vi "Fuzzy_Output.vi"() -> ()   [LabVIEW 2016]
panel:
  in  "OK Button":bool
  in  "stop":bool
  in  "Membership Function 3":dbl[](array[numeric])
  in  "Membership Function 2":dbl[](array[numeric])
  in  "Membership Function 1":dbl[](array[numeric])
  out "XY Graph":cluster{"Array":dbl[], dbl[]}[](graph)
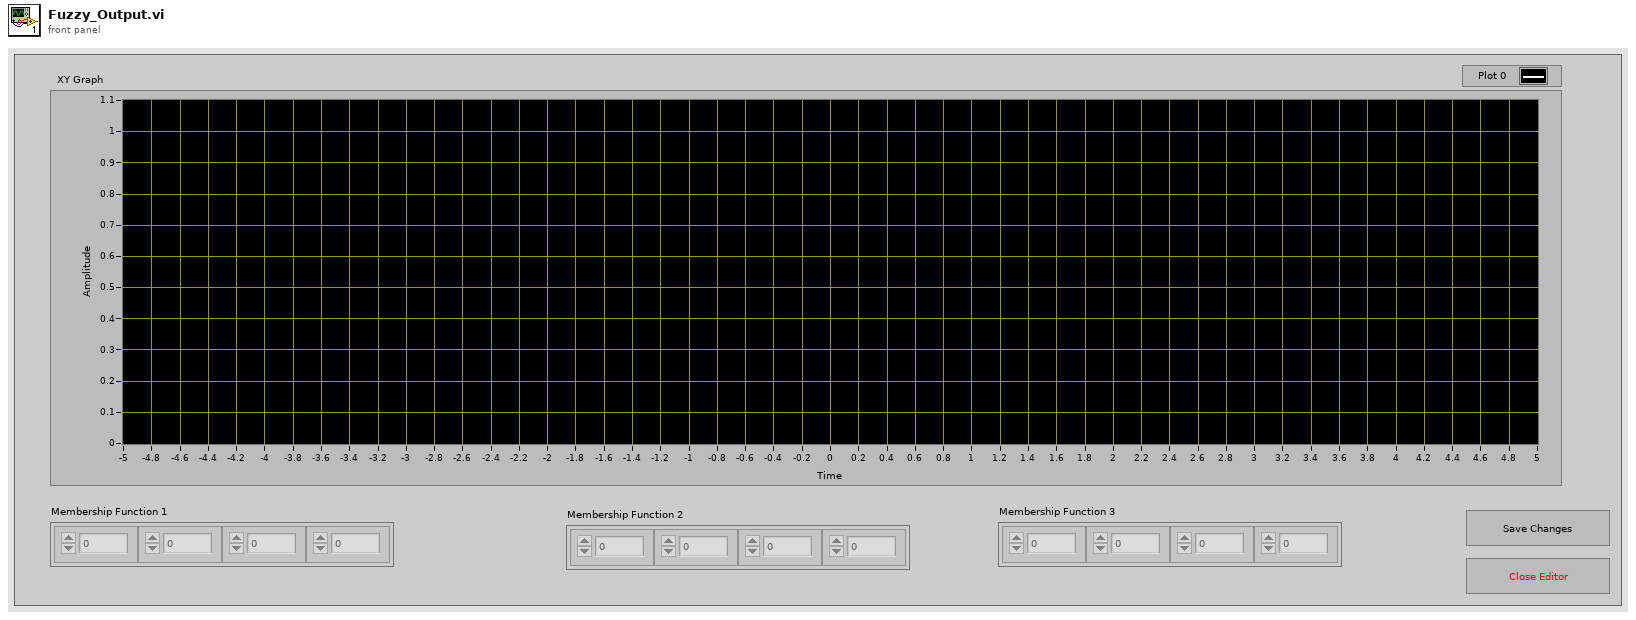
[diagram p1: front panel]
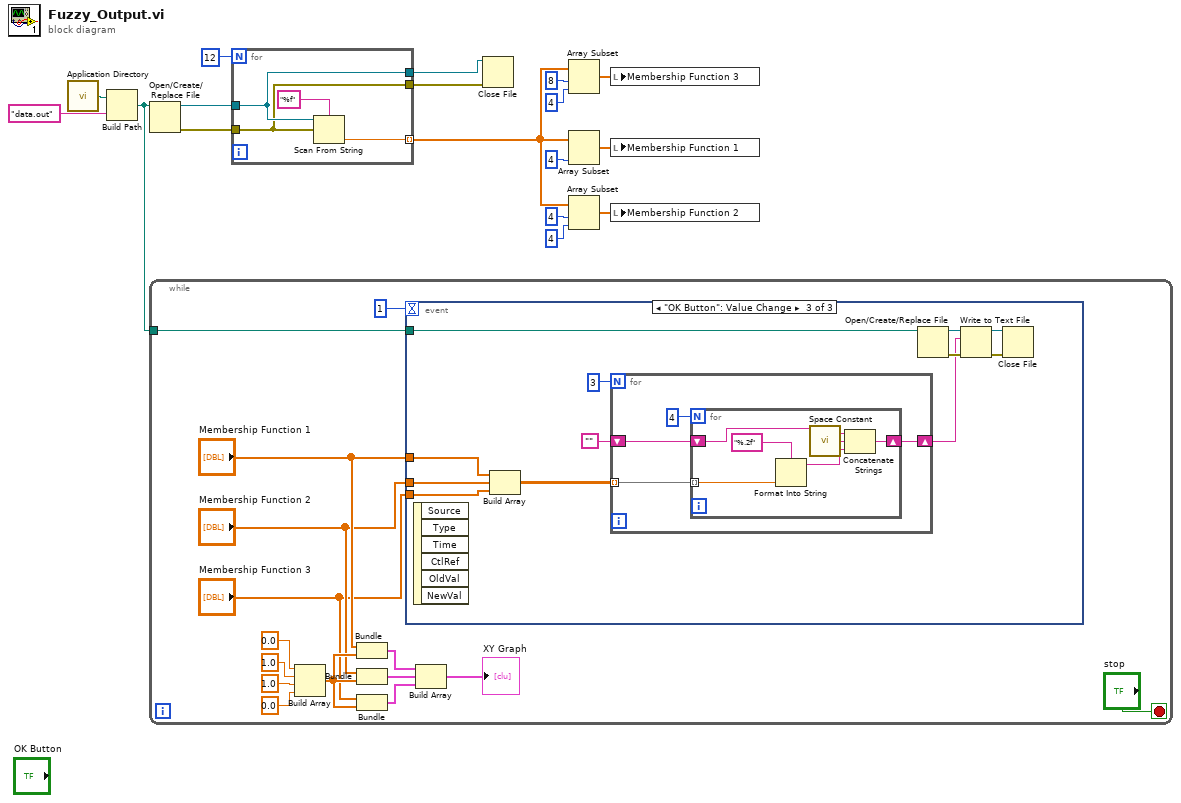
[diagram p0: block diagram]
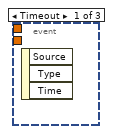
[diagram p2: hidden frame]
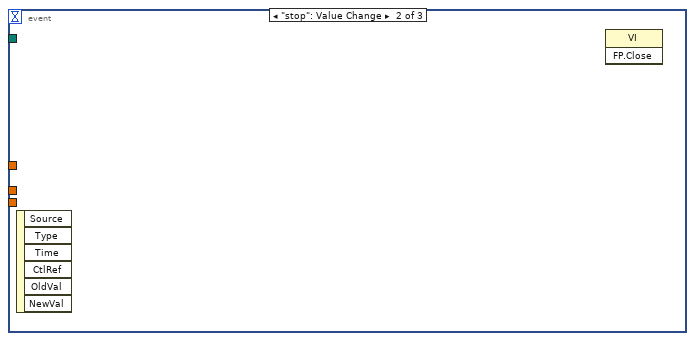
[diagram p3: hidden frame]
diagram:
  n1 = call <vilib>:"Application Directory.vi"() -> ("Application Directory"=w16:path)
  n2 = Build Path(base path=w16, name or relative path="data.out") -> (appended path=w1:path)
  n3 = Open/Create/Replace File(file path (use dialog)=w1) -> (refnum out=w14:refnum<file>, error out=w13:errorcluster)  [unwired: 5 in, 1 out]
  n4 = while {
    tunnel: w1 -> [w18]
    stop <- "stop" stop-if-true
    n5 = Build Array(0.0 ("element"), 1.0 ("element"), 1.0 ("element"), 0.0 ("element")) -> (w24:dbl[])
    n6 = Bundle("Membership Function 1"="Membership Function 1", w24) -> (w32:cluster{"Membership Function 1":dbl[], dbl[]})  [unwired: 1 in]
    n7 = Bundle("Membership Function 2"="Membership Function 2", w24) -> (w31:cluster{"Membership Function 2":dbl[], dbl[]})  [unwired: 1 in]
    n8 = Bundle("Membership Function 3"="Membership Function 3", w24) -> (w30:cluster{"Membership Function 3":dbl[], dbl[]})  [unwired: 1 in]
    n9 = event shown="[2] \"OK Button\": Value Change" {
      selector: _ -> [_ _ _]
      dyn-events: _ -> [_ _ _]
      timeout: 1 -> [_ _ _]
      tunnel: "Membership Function 1" -> [_ _ w36]
      tunnel: "Membership Function 2" -> [_ _ w35]
      tunnel: "Membership Function 3" -> [_ _ w34]
      tunnel: w18 -> [_ _ w33]
      event Timeout {
        n10 = event-data() -> ()  [unwired: 1 in, 3 out]
      }
      event "stop": Value Change {
        n11 = event-data() -> ()  [unwired: 1 in, 6 out]
        n12 = invoke class="VI" method="FP.Close"() -> ()  [unwired: 3 in, 3 out]
      }
      event "OK Button": Value Change {
        n13 = event-data() -> ()  [unwired: 1 in, 6 out]
        n14 = Build Array(w36, w35, w34) -> (w38:dbl[][])
        n15 = for {
          N: 3 -> [_]
          tunnel: w38 -> [w47] mode=indexing
          shift-right: [w46] -> w40
          shift-left: "" -> [w45]
          n16 = for {
            N: 4 -> [_]
            tunnel: w47 -> [w49] mode=indexing
            shift-right: [w53] -> w46
            shift-left: w45 -> [w52]
            n17 = Format Into String(format string="%.2f", w49) -> (resulting string=w50:string)  [unwired: 2 in, 1 out]
            n18 = call <vilib>:"Space Constant.vi"() -> ("String"=w51:string)
            n19 = Concatenate Strings(w52, w51, w50) -> (w53:string)
          }
        }
        n20 = Open/Create/Replace File(file path (use dialog)=w33) -> (refnum out=w41:refnum<file>, error out=w42:errorcluster)  [unwired: 5 in, 1 out]
        n21 = Write to Text File(file (use dialog)=w41, text=w40, error in=w42) -> (refnum out=w43:refnum<file>, error out=w44:errorcluster)  [unwired: 1 in, 1 out]
        n22 = Close File(refnum=w43, error in=w44) -> ()  [unwired: 2 out]
      }
    }
    n23 = Build Array(w32, w31, w30) -> (→"XY Graph":cluster{"Membership Function 3":dbl[], dbl[]}[])
  }
  n24 = for {
    N: 12 -> [_]
    tunnel: w14 -> [w56]
    tunnel: w13 -> [w55]
    tunnel: [w57] -> w6 mode=indexing
    tunnel: [w56] -> w3
    tunnel: [w55] -> w2
    n25 = Scan From String("%f" ("format string"), w56, w55) -> (output 1=w57:dbl)  [unwired: 1 in, 2 out]
  }
  n26 = Close File(refnum=w3, error in=w2) -> ()  [unwired: 2 out]
  n27 = Array Subset(array=w6, index=8, length=4) -> (w7:dbl[])
  n28 = Array Subset(array=w6, length=4) -> (w11:dbl[])  [unwired: 1 in]
  n29 = Array Subset(array=w6, index=4, length=4) -> (w10:dbl[])
  n30 = local write "Membership Function 3"(w7) -> ()
  n31 = local write "Membership Function 1"(w11) -> ()
  n32 = local write "Membership Function 2"(w10) -> ()
